vi "Send Message.vi"(8 "error in (no error)":errorcluster, 10 "Write Request":T1, 11 "Connection Handler in":refnum<class "Connection Handler.lvclass">) -> (0 "error out":errorcluster, 3 "Connection Handler out":refnum<class "Connection Handler.lvclass">)   [LabVIEW 2019, in "Network Interface.lvlib" / "Connection Handler.lvclass"]
uses:
  <vilib>/gpm_packages/@cs/Network-Sink/Source/Network Interface/Connection Handler/Connection Handler.lvclass
  <vilib>/gpm_packages/@cs/Network-Sink/Source/Network Interface/Connection Handler/Synchronous Write Request.ctl
  <vilib>/gpm_packages/@cs/Network-Sink/Source/Network Interface/Connection Handler/Connection Handler.lvclass/Connection Handler.ctl
  <vilib>/gpm_packages/@cs/Network-Sink/Source/Network Interface/IConnection/IConnection.lvclass
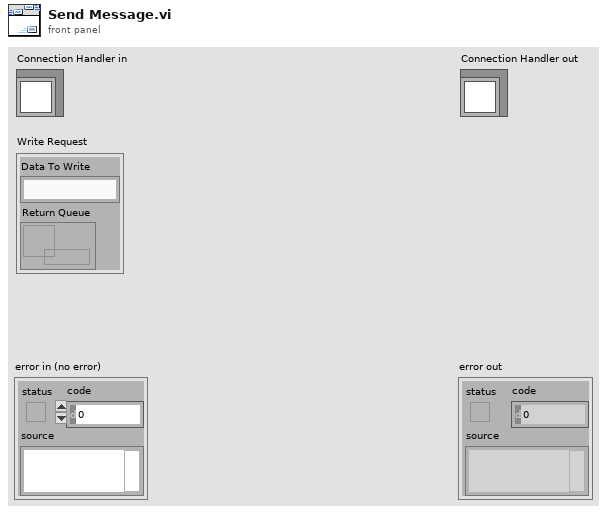
[diagram p1: front panel]
types:
  T1 = typedef "Network Interface.lvlib/Connection Handler.lvclass/Synchronous Write Request.ctl" = cluster{"Data To Write":string, "Return Queue":refnum<queue>}
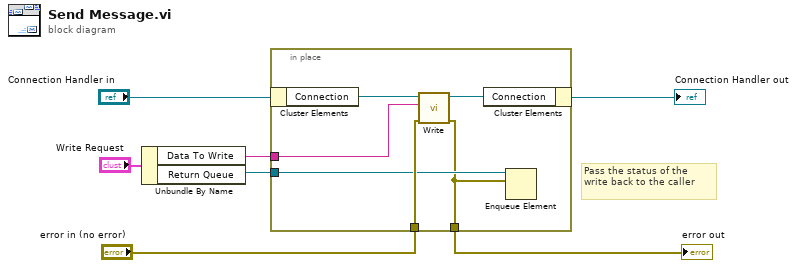
[diagram p0: block diagram]
diagram:
  # "Pass the status of the write back to the caller"
  n1 = Unbundle By Name("Write Request") -> ("Data To Write"=w5:string, "Return Queue"=w4:refnum<queue>)
  n2 = in-place {
    in-place-border: "error in (no error)" -> [w13]
    in-place-border: w5 -> [w8]
    in-place-border: w4 -> [w12]
    in-place-border: [w11] -> w3
    n3 = in-place-cluster #1("Connection Handler in") -> ("Connection"=w10:refnum<class "IConnection.lvclass">)
    n4 = call-dynamic "Write.vi"("error in (no error)"=w13, "Data to Write"=w8, "IConnection in"=w10) -> ("error out"=w11:errorcluster, "IConnection out"=w9:refnum<class "IConnection.lvclass">)  [unwired: 7 in]
    n5 = in-place-cluster #1("Connection"=w9) -> (→"Connection Handler out":refnum<class "Connection Handler.lvclass">)
    n6 = Enqueue Element(queue=w12, element=w11) -> ()  [unwired: 2 in, 3 out]
  }
  "error out" <- w3
